vi "Check SysDef for VCOM Signal.vi"(8 "error in (no error)":errorcluster, 10 "VCOM Signal Map In":map{string, T1}(c390), 11 "System Definition File Path":path=path "C:/Users/Nick/Desktop/VCOM Config System Definition Utility/VeriStand Example Project/Example Project/Example Project.nivssdf") -> (0 "error out":errorcluster, 2 "Deprecated Signal GUIDs":u64[](array[numeric]), 3 "Signals Not Found in new VCOM Config":string[](array[string]))   [LabVIEW 2025]
uses:
  <vilib>/Vehicle Communication Toolkit/TypDefs/RBS Signal.ctl
  NationalInstruments.VeriStand.SystemDefinitionAPI
  <vilib>/NI/NI VeriStand Advanced SysDef API/_SubVIs/SysDef.Search.GUIDs.vi
  NationalInstruments.VeriStand.SystemStorage
  <vilib>/NI/NI VeriStand Advanced SysDef API/SysDef API/Advanced System Definition.lvlib
  <vilib>/Vehicle Communication Toolkit/Vehicle Communication Toolkit.lvlib
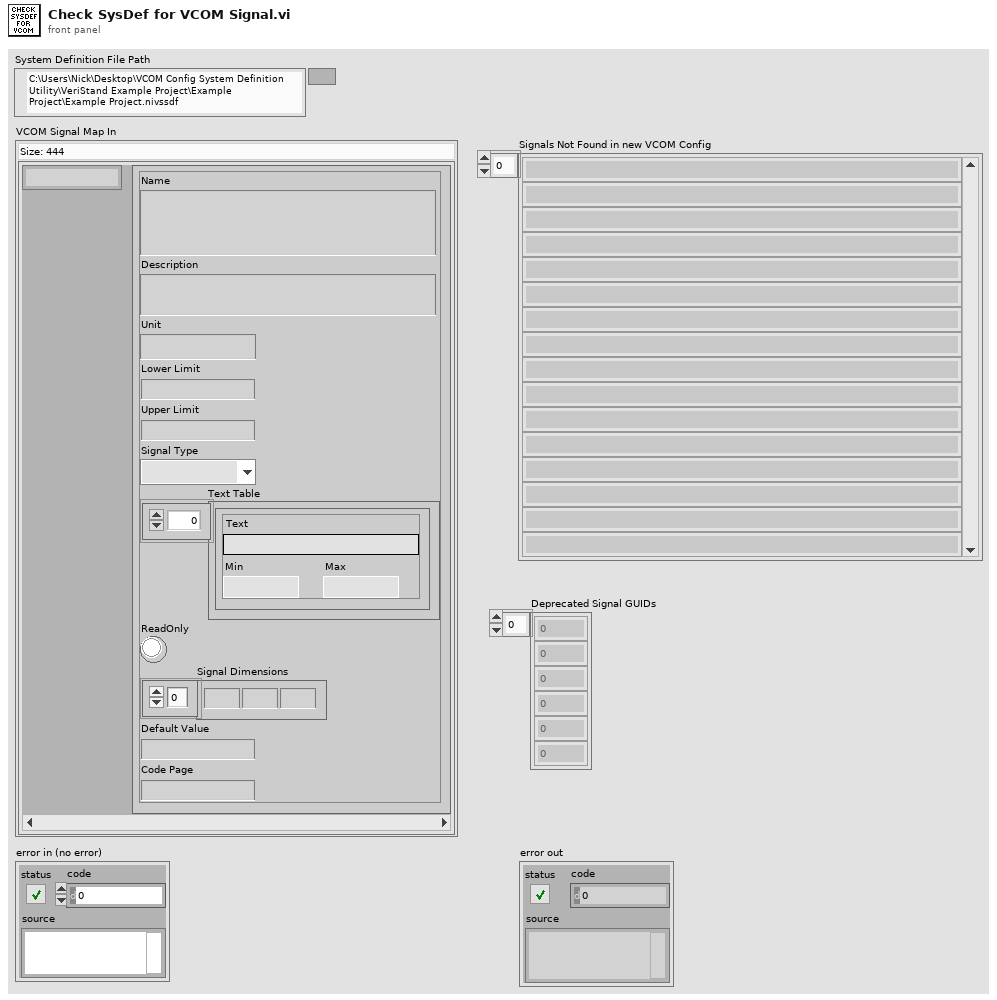
[diagram p1: front panel]
types:
  T1 = typedef "Vehicle Communication Toolkit.lvlib/RBS Signal.ctl" = cluster{"Name":string, "Description":string, "Unit":string, "Lower Limit":dbl, "Upper Limit":dbl, "Signal Type":enum32{"RE_BOOL", "RE_UINT8", "RE_INT8", "RE_UINT16", "RE_INT16", "RE_UINT32", "RE_INT32", "RE_UINT64", "RE_INT64", "RE_FLOAT32", "RE_FLOAT64", "RE_TEXT"}, "Text Table":cluster{"Text":string, "Min":dbl, "Max":dbl}[], "ReadOnly":bool, "Signal Dimensions":u32[], "Default Value":dbl, "Code Page":u32}
  T2 = typedef "Custom Device API.lvlib/Custom Device Pointer.ctl" = refnum<k24>
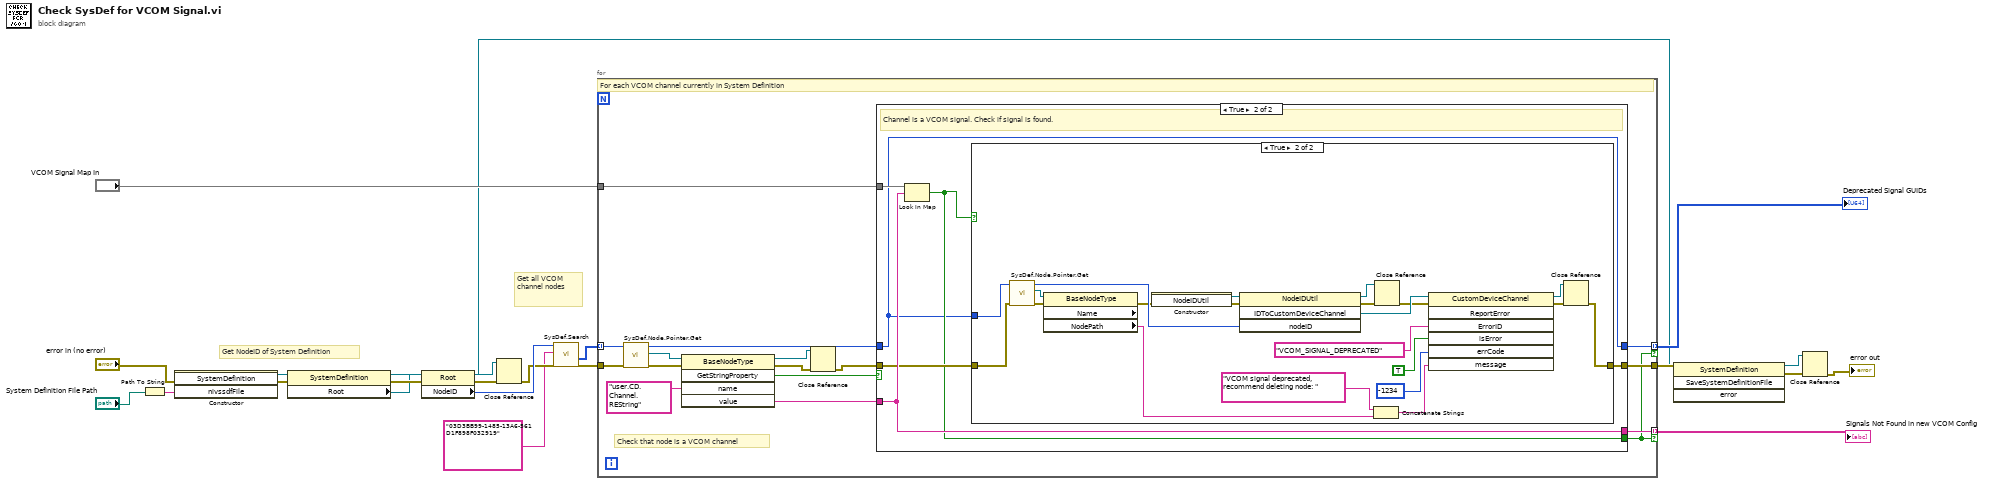
[diagram p0: block diagram]
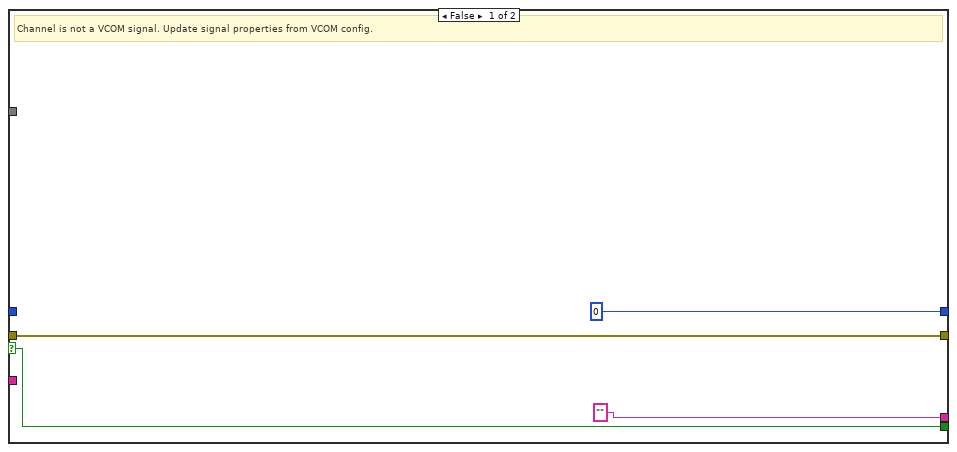
[diagram p2: hidden frame]
diagram:
  # "Get all VCOM channel nodes"
  # "Get NodeID of System Definition"
  n1 = Path To String(path="System Definition File Path") -> (string=w20:string)
  n2 = constructor class="SystemDefinition"(error in="error in (no error)", "nivssdfFile"=w20) -> (reference out=w18:refnum<k24>, error out=w19:errorcluster)  [unwired: 2 in, 2 out]
  n3 = property class="SystemDefinition"(reference=w18, error in=w19) -> (reference out=w4:refnum<k24>, error out=w16:errorcluster, "Root"=w8:refnum<k24>)
  n4 = property class="Root"(reference=w8, error in=w16) -> (reference out=w13:refnum<k24>, error out=w14:errorcluster, "NodeID"=w15:u64)
  n5 = Close Reference(reference=w13, error in (no error)=w14) -> (error out=w12:errorcluster)
  n6 = call-poly <vilib>:"SysDef.Search.vi"("error in (no error)"=w12, "GUID"="03D3BB99-1485-13A6-561D1F898F032919", "nodeID"=w15) -> ("error out"=w22:errorcluster, "Values Out"=w21:u64[])  [unwired: 5 in, 2 out]
  n7 = for {
    tunnel: w21 -> [w32] mode=indexing
    tunnel: "VCOM Signal Map In" -> [w34]
    tunnel: w22 -> [w36]
    tunnel: [w30] -> w5
    tunnel: [w28] -> w7 mode=indexing if=w26
    tunnel: [w27] -> w6 mode=indexing if=w26
    # "Check that node is a VCOM channel"
    # "For each VCOM channel currently in System Definition"
    n8 = call <vilib>:"SysDef.Node.Pointer.Get.vi"("error in (no error)"=w36, "nodeID"=w32) -> ("error out"=w35:errorcluster, "Node Pointer"=w38:T2, "nodeID out"=w31:u64)  [unwired: 6 in, 1 out]
    n9 = invoke class="BaseNodeType" method="GetStringProperty"(reference=w38, error in=w35, "name"="user.CD.Channel.REString") -> (reference out=w24:T2, error out=w25:errorcluster, "GetStringProperty"=w29:bool, "value"=w33:string)  [unwired: 2 in, 1 out]
    n10 = Close Reference(reference=w24, error in (no error)=w25) -> (error out=w23:errorcluster)
    n11 = case shown="True" w29 {
      selector: w29 -> [w40 _]
      tunnel: w34 -> [_ w48]
      tunnel: w33 -> [_ w47]
      tunnel: w23 -> [w42 w46]
      tunnel: w31 -> [_ w44]
      tunnel: [w42 w43] -> w30
      tunnel: ["" ("value") w47] -> w28
      tunnel: [w40 w45] -> w26
      tunnel: [u64 0 ("nodeID out") w44] -> w27
      frame False {
        # "Channel is not a VCOM signal. Update signal properties from VCOM config."
      }
      frame True {
        # "Channel is a VCOM signal. Check if signal is found."
        n12 = Look In Map(map=w48, key=w47) -> (key not found?=w45:bool)  [unwired: 1 in, 1 out]
        n13 = case shown="True" w45 {
          tunnel: w46 -> [w49 w70]
          tunnel: w44 -> [_ w69]
          tunnel: [w49 w68] -> w43
          frame False {
          }
          frame True {
            n14 = call <vilib>:"SysDef.Node.Pointer.Get.vi"("error in (no error)"=w70, "nodeID"=w69) -> ("error out"=w64:errorcluster, "Node Pointer"=w65:T2, "nodeID out"=w63:u64)  [unwired: 6 in, 1 out]
            n15 = property class="BaseNodeType" props=["Name", "NodePath"](reference=w65, error in=w64) -> (error out=w57:errorcluster, "NodePath"=w51:string)  [unwired: 2 out]
            n16 = constructor class="NodeIDUtil"(error in=w57) -> (reference out=w56:refnum<k24>, error out=w58:errorcluster)  [unwired: 2 in, 1 out]
            n17 = invoke class="NodeIDUtil" method="IDToCustomDeviceChannel"(reference=w56, error in=w58, "nodeID"=w63) -> (reference out=w55:refnum<k24>, error out=w54:errorcluster, "IDToCustomDeviceChannel"=w59:refnum<k24>)  [unwired: 1 in, 1 out]
            n18 = Concatenate Strings("VCOM signal deprecated, recommend deleting node: " ("ErrorID"), w51) -> (w50:string)
            n19 = Close Reference(reference=w55, error in (no error)=w54) -> (error out=w53:errorcluster)
            n20 = invoke class="CustomDeviceChannel" method="ReportError"(reference=w59, error in=w53, "ErrorID"="VCOM_SIGNAL_DEPRECATED", "isError"=TRUE, "errCode"=-1234, "message"=w50) -> (reference out=w66:refnum<k24>, error out=w67:errorcluster)  [unwired: 1 in, 5 out]
            n21 = Close Reference(reference=w66, error in (no error)=w67) -> (error out=w68:errorcluster)
          }
        }
      }
    }
  }
  "Signals Not Found in new VCOM Config" <- w7
  "Deprecated Signal GUIDs" <- w6
  n22 = invoke class="SystemDefinition" method="SaveSystemDefinitionFile"(reference=w4, error in=w5) -> (reference out=w2:refnum<k24>, error out=w3:errorcluster)  [unwired: 2 in, 2 out]
  n23 = Close Reference(reference=w2, error in (no error)=w3) -> (error out=→"error out":errorcluster)
